vi "Core.vi"(8 "error in (no error)":errorcluster, 9 "CurWeek(0)":i32, 10 "ExcusePath":path, 11 "CalAttendance in":refnum<class "CalAttendance.lvclass">) -> (0 "error out":errorcluster, 3 "CalAttendance out":refnum<class "CalAttendance.lvclass">)   [LabVIEW 2015, in "CalAttendance.lvclass"]
uses:
  CalAttendance.lvclass
  Models/ExcelReader/ExcelReader.lvclass
  CalAttendance.lvclass/CalAttendance.ctl
  Member_Actor/MemberTable/TimeTable.lvclass
  ExcuseNotes/ExcuseNotesHandler.lvclass
  Models/Attendance Record/AttendRecord.lvclass
  Models/MemberAttendance/MemberAttendance.lvclass/MemberAttendance.ctl
  ExcuseNotes/ExcuseNotesHandler.lvclass/ExcuseNotesHandler.ctl
  Models/Attendance Record/AttendRecord.lvclass/AttendRecord.ctl
  Setting/g_setting.vi
  Models/MemberAttendance/MemberAttendance.lvclass
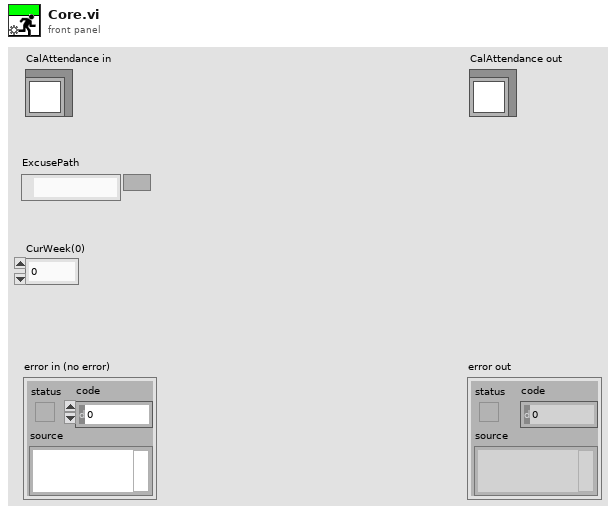
[diagram p1: front panel]
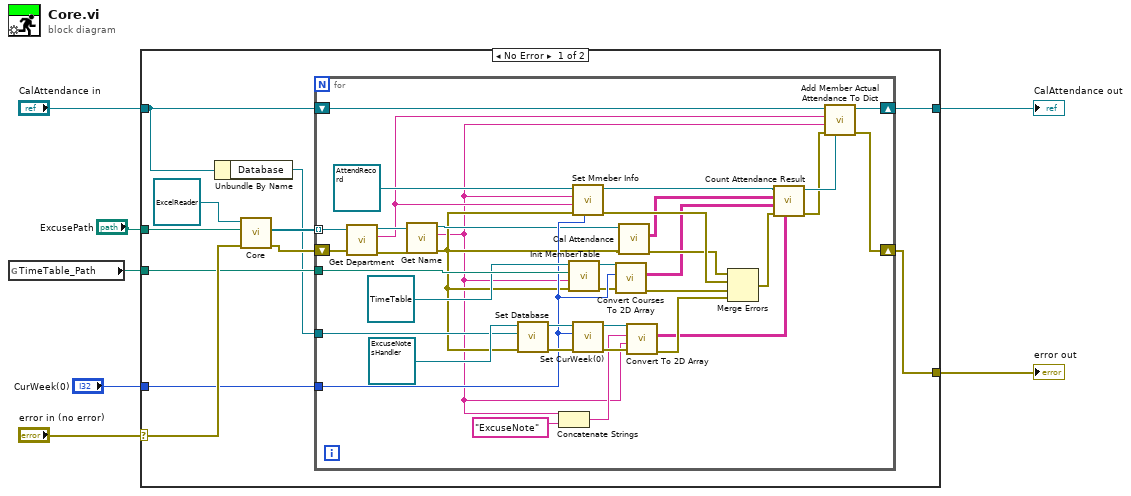
[diagram p0: block diagram]
diagram:
  n1 = global read "g_setting.vi" "TimeTable_Path"() -> (w2:path)
  n2 = case shown="No Error" "error in (no error)" {
    selector: "error in (no error)" -> [w16 w56]
    tunnel: [w12 w56] -> w6
    tunnel: [w8 w55] -> w4
    tunnel: "CalAttendance in" -> [w9 w55]
    tunnel: "ExcusePath" -> [w17 _]
    tunnel: w2 -> [w13 _]
    tunnel: "CurWeek(0)" -> [w10 _]
    frame No Error {
      n3 = Unbundle By Name(w9) -> ("Database"=w11:refnum<class "Database.lvclass">)
      n4 = call "Core.vi"("error in (no error)"=w16, "Path"=w17, "ExcelReader in"=refnum<class "ExcelReader.lvclass"> refnum ("Admin_Actor.lvlib:ExcelReader.lvclass")) -> ("error out"=w14:errorcluster, "MemberAttendance"=w15:refnum<class "MemberAttendance.lvclass">[])  [unwired: 6 in, 1 out]
      n5 = for {
        tunnel: w15 -> [w46] mode=indexing
        tunnel: w13 -> [w54]
        shift-right: [w39] -> w12
        shift-left: w14 -> [w45]
        tunnel: w11 -> [w49]
        tunnel: w10 -> [w37]
        shift-right: [w40] -> w8
        shift-left: w9 -> [w42]
        n6 = call "Get Department.vi"("error in (no error)"=w45, "MemberAttendance in"=w46) -> ("error out"=w43:errorcluster, "Department(\"\")"=w41:string, "MemberAttendance out"=w44:refnum<class "MemberAttendance.lvclass">)  [unwired: 7 in]
        n7 = call "Get Name.vi"("error in (no error)"=w43, "MemberAttendance in"=w44) -> ("error out"=w31:errorcluster, "Name(\"\")"=w19:string, "MemberAttendance out"=w32:refnum<class "MemberAttendance.lvclass">)  [unwired: 7 in]
        n8 = call "Set Database.vi"("error in (no error)"=w31, "Database"=w49, "ExcuseNotes in"=refnum<class "ExcuseNotesHandler.lvclass"> refnum ("Admin_Actor.lvlib:ExcuseNotes.lvclass")) -> ("error out"=w52:errorcluster, "ExcuseNotes out"=w51:refnum<class "ExcuseNotesHandler.lvclass">)  [unwired: 7 in]
        n9 = Concatenate Strings(w19, "ExcuseNote" ("string")) -> (w20:string)
        n10 = call "Init MemberTable.vi"("error in (no error)"=w31, "SheetName(\"\")"=w19, "Path"=w54, "TimeTable in"=refnum<class "TimeTable.lvclass"> refnum) -> ("error out"=w36:errorcluster, "TimeTable out"=w38:refnum<class "TimeTable.lvclass">)  [unwired: 6 in]
        n11 = call "Set Mmeber Info.vi"("Week(0)"=w37, "error in (no error)"=w31, "Department(\"\")"=w41, "Name(\"\")"=w19, "AttendRecord in"=refnum<class "AttendRecord.lvclass"> refnum ("AttendRecord.lvclass")) -> ("error out"=w47:errorcluster, "AttendRecord out"=w28:refnum<class "AttendRecord.lvclass">)  [unwired: 5 in]
        n12 = call "Set CurWeek(0).vi"("error in (no error)"=w52, "CurWeek(0)"=w37, "ExcuseNotesHandler in"=w51) -> ("error out"=w34:errorcluster, "ExcuseNotesHandler out"=w35:refnum<class "ExcuseNotesHandler.lvclass">)  [unwired: 7 in]
        n13 = call "Convert Courses To 2D Array.vi"("error in (no error)"=w36, "CurWeek(0)"=w37, "TimeTable in"=w38) -> ("error out"=w30:errorcluster, "Array"=w23:string[][])  [unwired: 6 in, 1 out]
        n14 = call "Cal Attendance.vi"("error in (no error)"=w31, "MemberAttendance in"=w32) -> ("error out"=w29:errorcluster, "Attendance Result(\"\")"=w24:string[][])  [unwired: 7 in, 1 out]
        n15 = call "Convert To 2D Array.vi"("error in (no error)"=w34, "Name"=w19, "TableName"=w20, "ExcuseNotesHandler"=w35) -> ("error out"=w33:errorcluster, "2D Array"=w22:string[][])  [unwired: 5 in, 1 out]
        n16 = Merge Errors(w29, w47, w30, w33) -> (w25:errorcluster)
        n17 = call "Count Attendance Result.vi"("ExcuseNotes(\"\")"=w22, "error in (no error)"=w25, "TimeTables(\"\")"=w23, "Calendances(\"\")"=w24, "AttendRecord.lvclass"=w28) -> ("error out"=w26:errorcluster, "AttendRecord.lvclass Out"=w27:refnum<class "AttendRecord.lvclass">)  [unwired: 5 in]
        n18 = call "Add Member Actual Attendance To Dict.vi"("AttendRecord.lvclass"=w27, "error in (no error)"=w26, "Name(\"\")"=w19, "Department(\"\")"=w41, "CalAttendance in"=w42) -> ("error out"=w39:errorcluster, "CalAttendance out"=w40:refnum<class "CalAttendance.lvclass">)  [unwired: 5 in]
      }
    }
    frame Error {
    }
  }
  "error out" <- w6
  "CalAttendance out" <- w4
